vi "Write Value (variant).vi"(8 "error in (no error)":errorcluster, 10 "Variant":variant, 11 "Float D Element in":refnum<class "Float D Element.lvclass">) -> (0 "error out":errorcluster, 3 "Float D Element out":refnum<class "Float D Element.lvclass">)   [LabVIEW 2018, in "D Datagrid Library.lvlib" / "Float D Element.lvclass"]
uses:
  Float D Element.lvclass
  Float D Element.lvclass/Float D Element.ctl
  Write Value.vi
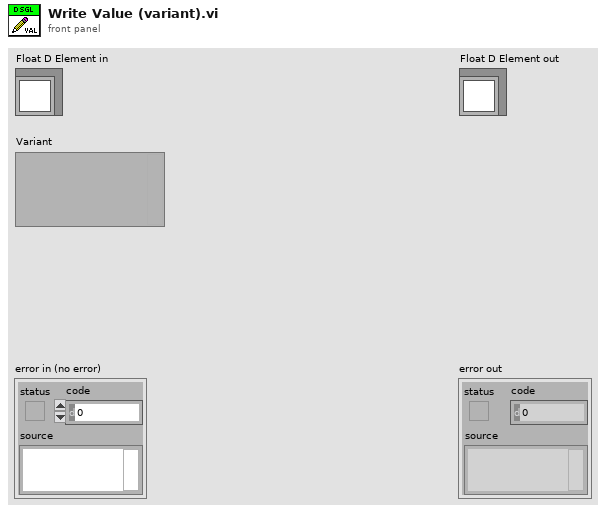
[diagram p1: front panel]
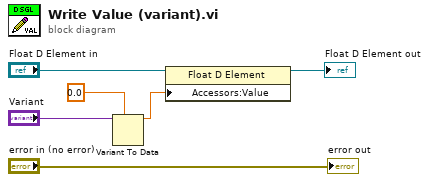
[diagram p0: block diagram]
diagram:
  n1 = Variant To Data(type=sgl 0.0 ("Value"), Variant="Variant") -> (data=w2:sgl)  [unwired: 1 in, 1 out]
  n2 = property class="Float D Element"(reference="Float D Element in", "Accessors:Value"=w2) -> (reference out=→"Float D Element out":refnum<class "Float D Element.lvclass">)  [unwired: 1 in, 1 out]
  "error out" <- "error in (no error)"
